vi "SQL_CloseIncidence.vi"(0 "ConnectionDSN":string, 1 "TableName":string, 2 "IncidenceID":string, 3 "ToolCribFolio":string, 4 "EWOFolio":string, 5 "Comments":string) -> ()   [LabVIEW 2017]
uses:
  <vilib>/addons/database/Connection.llb/DB Tools Open Connec (String).vi
  <vilib>/addons/database/Connection.llb/Conn Execute.vi
  <vilib>/addons/database/Recordset.llb/Rec Fetch Recordset Data (R).vi
  <vilib>/addons/database/_DB Variant To Data/Database Variant To Data.xnode
  <vilib>/addons/database/NI_Database_API.lvlib
panel:
  out "error out":errorcluster
  # "This VI Updates the hour when the machine starts production and records the downtime in minutes\ninto the database"
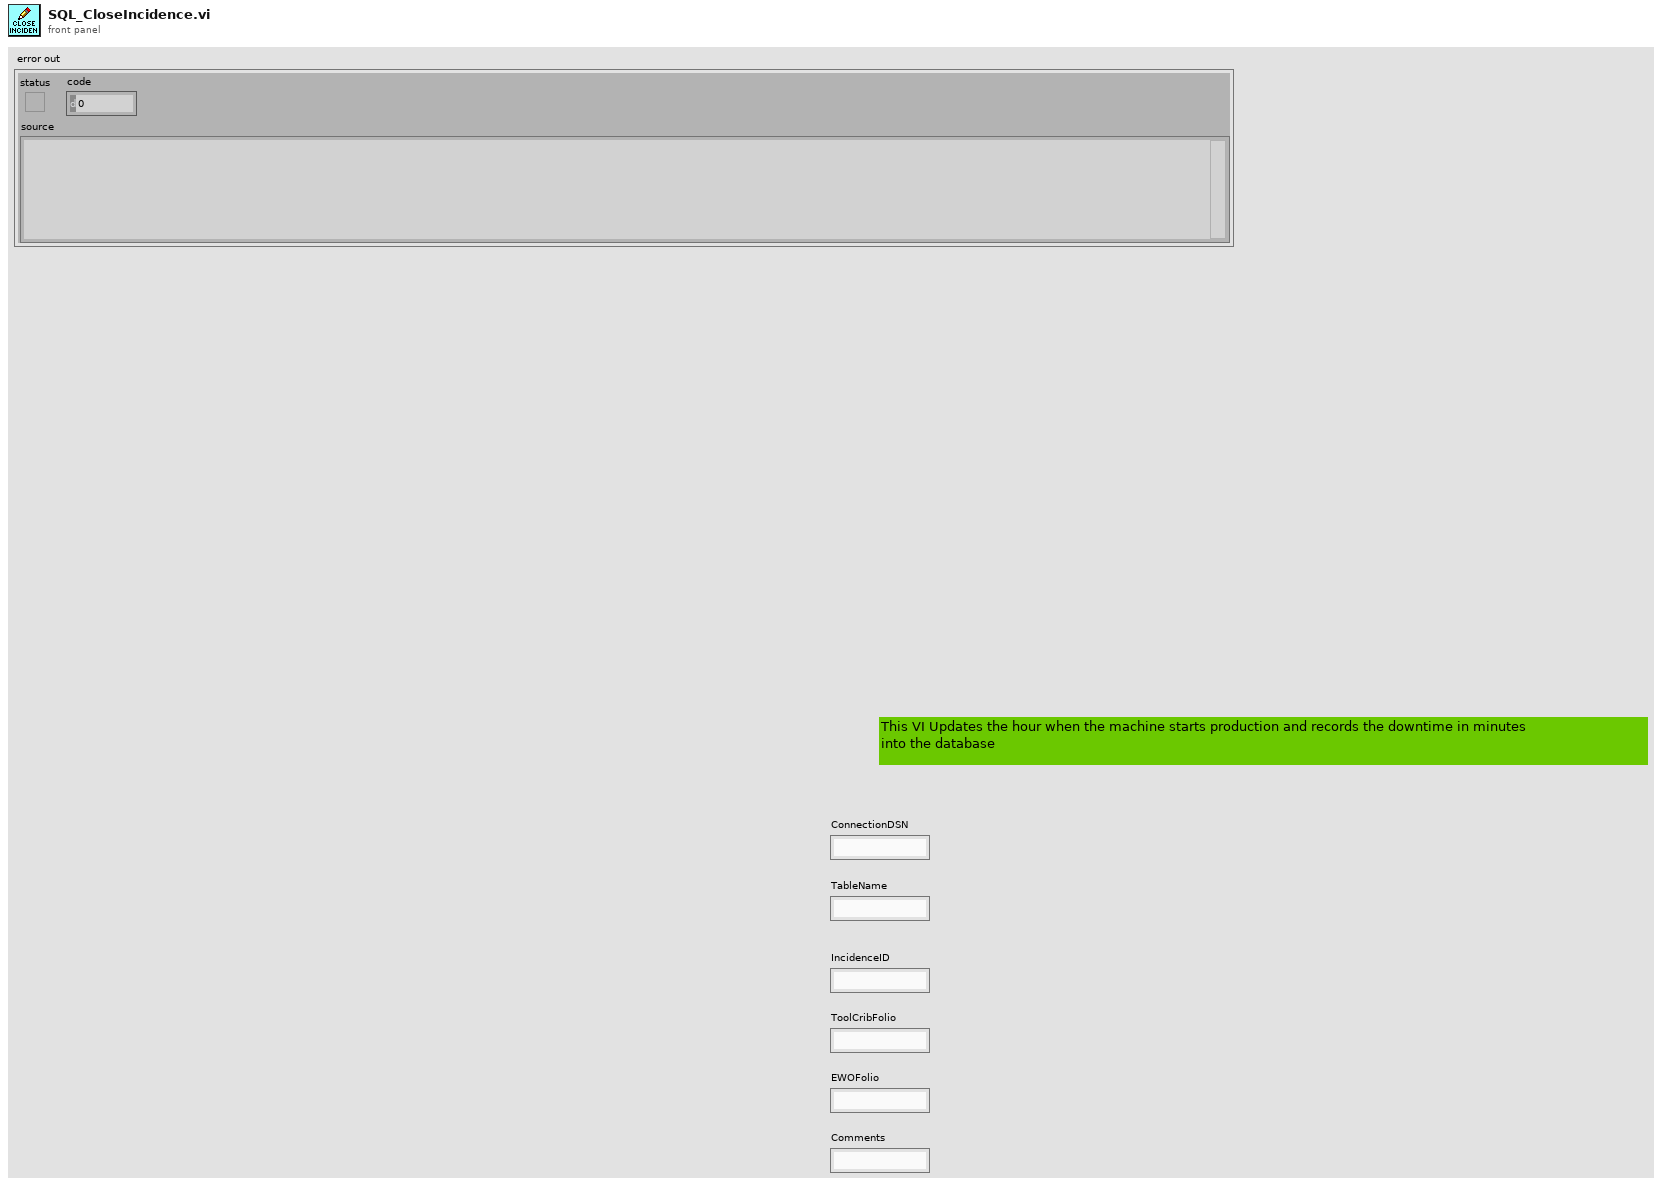
[diagram p1: front panel]
types:
  T1 = typedef "NI_Database_API.lvlib/Conn ObjectReference.ctl" = refnum<k1>
  T2 = typedef "NI_Database_API.lvlib/Rec ObjectReference.ctl" = refnum<k1>
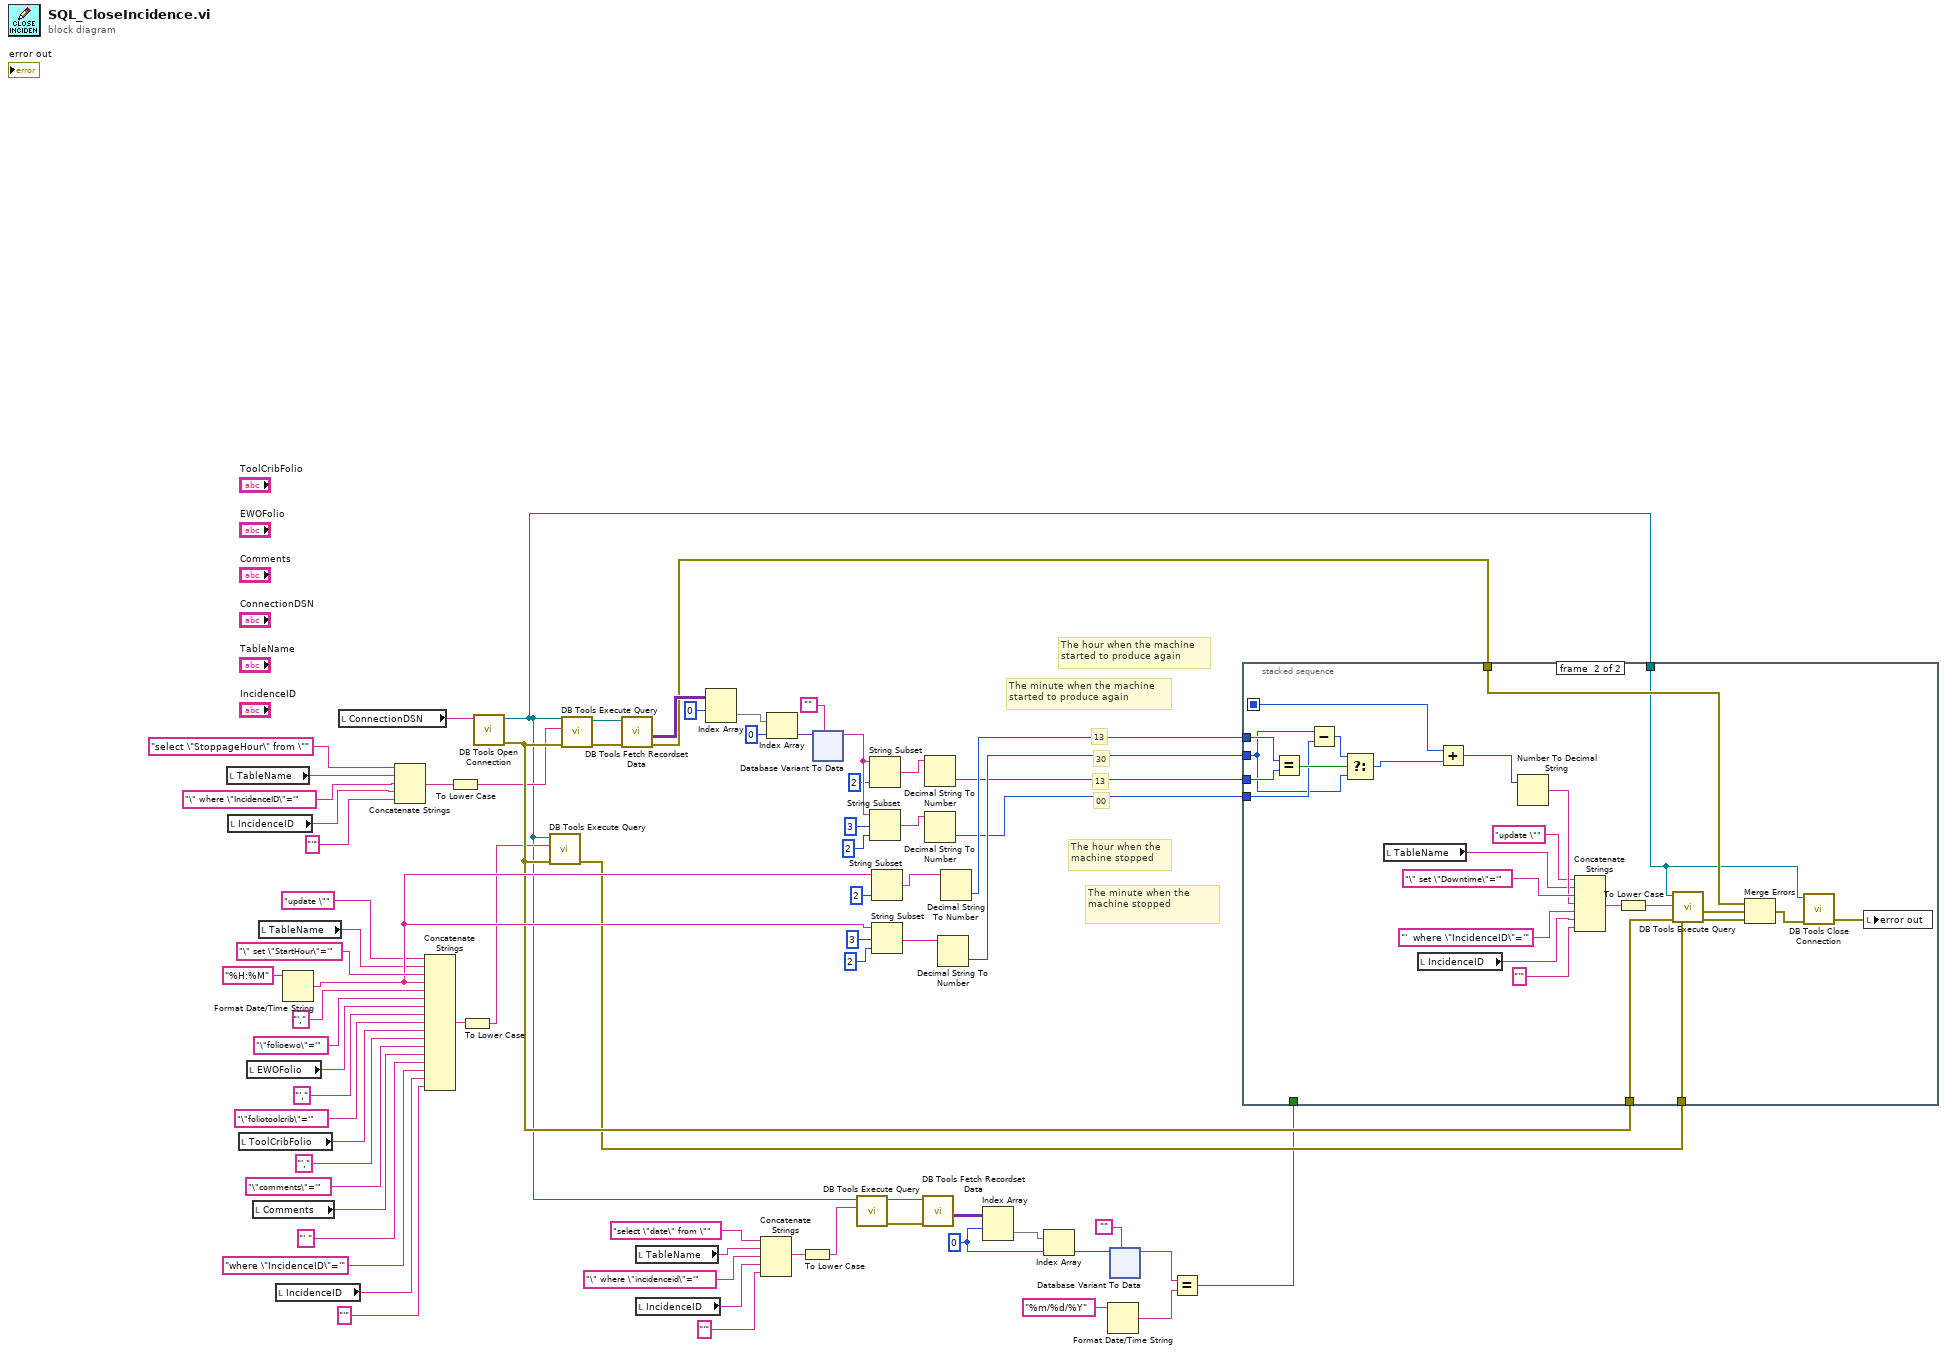
[diagram p0: block diagram]
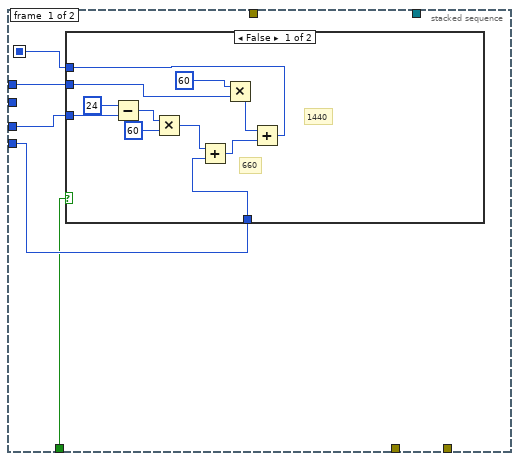
[diagram p2: hidden frame]
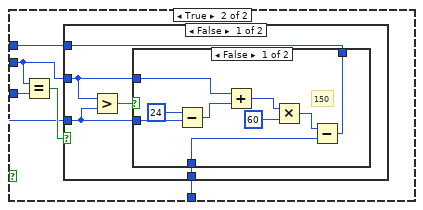
[diagram p3: hidden frame]
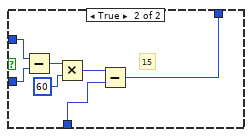
[diagram p4: hidden frame]
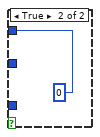
[diagram p5: hidden frame]
diagram:
  w7 = 0 ("index (row)")
  # "The hour when the machine\nstarted to produce again"
  # "The minute when the machine\nstarted to produce again"
  # "The minute when the\nmachine stopped"
  # "The hour when the\nmachine stopped"
  # "30"
  # "13"
  # "13"
  # "00"
  n1 = local read "TableName"() -> (w40:string)
  n2 = local read "IncidenceID"() -> (w38:string)
  n3 = local read "ToolCribFolio"() -> (w31:string)
  n4 = local read "EWOFolio"() -> (w33:string)
  n5 = local read "Comments"() -> (w28:string)
  n6 = local read "TableName"() -> (w43:string)
  n7 = local read "IncidenceID"() -> (w25:string)
  n8 = Format Date/Time String(time format string (%c)="%H:%M") -> (date/time string=w56:string)  [unwired: 2 in]
  n9 = local read "ConnectionDSN"() -> (w42:string)
  n10 = Concatenate Strings("select \"StoppageHour\" from \"" ("SQL query"), w40, "\" where \"IncidenceID\"='" ("SQL query"), w38, "'" ("SQL query")) -> (w21:string)
  n11 = Concatenate Strings("update \"" ("SQL query"), w43, "\" set \"StartHour\"='" ("SQL query"), w56, "',", "\"folioewo\"='" ("SQL query"), w33, "',", "\"foliotoolcrib\"='" ("SQL query"), w31, "',", "\"comments\"='" ("SQL query"), w28, "' ", "where \"IncidenceID\"='", w25, "'") -> (w23:string)
  n12 = To Lower Case(string=w21) -> (all lower case string=w20:string)
  n13 = To Lower Case(string=w23) -> (all lower case string=w22:string)
  n14 = call-poly <vilib>:"DB Tools Open Connection.vi"("connection information"=w42) -> ("error out"=w47:errorcluster, "connection reference"=w19:T1)  [unwired: 7 in]
  n15 = call-poly <vilib>:"DB Tools Execute Query.vi"("error in (no error)"=w47, "SQL query"=w22, "connection reference"=w19) -> ("error out"=w46:errorcluster)  [unwired: 5 in, 1 out]
  n16 = call-poly <vilib>:"DB Tools Execute Query.vi"("error in (no error)"=w47, "SQL query"=w20, "connection reference"=w19) -> ("error out"=w73:errorcluster, "recordset reference"=w72:T2)  [unwired: 5 in]
  n17 = call-poly <vilib>:"DB Tools Fetch Recordset Data.vi"("error in (no error)"=w73, "recordset reference"=w72) -> ("error out"=w45:errorcluster, "recordset data"=w68:variant[][])  [unwired: 3 in, 1 out]
  n18 = local read "TableName"() -> (w17:string)
  n19 = local read "IncidenceID"() -> (w15:string)
  n20 = Index Array(array=w68, index (row)=0) -> (element=w70:variant[])  [unwired: 1 in]
  n21 = Concatenate Strings("select \"date\" from \"", w17, "\" where \"incidenceid\"='", w15, "'") -> (w13:string)
  n22 = Index Array(array=w70, index=0) -> (element=w67:variant)
  n23 = To Lower Case(string=w13) -> (all lower case string=w12:string)
  n24 = xnode "Database Variant To Data"("database variant"=w67, "type"="") -> ("data"=w65:string)  [unwired: 1 in, 1 out]
  n25 = call-poly <vilib>:"DB Tools Execute Query.vi"("SQL query"=w12, "connection reference"=w19) -> ("error out"=w10:errorcluster, "recordset reference"=w11:T2)  [unwired: 6 in]
  n26 = String Subset(string=w65, length (rest)=2 ("length (rest)")) -> (substring=w51:string)  [unwired: 1 in]
  n27 = String Subset(string=w65, offset (0)=3 ("length (rest)"), length (rest)=2 ("length (rest)")) -> (substring=w50:string)
  n28 = String Subset(string=w56, length (rest)=2 ("length (rest)")) -> (substring=w55:string)  [unwired: 1 in]
  n29 = String Subset(string=w56, offset (0)=3 ("length (rest)"), length (rest)=2 ("length (rest)")) -> (substring=w53:string)
  n30 = call-poly <vilib>:"DB Tools Fetch Recordset Data.vi"("error in (no error)"=w10, "recordset reference"=w11) -> ("recordset data"=w9:variant[][])  [unwired: 3 in, 2 out]
  n31 = Decimal String To Number(string=w51) -> (number=w49:i32)  [unwired: 2 in, 1 out]
  n32 = Decimal String To Number(string=w50) -> (number=w48:i32)  [unwired: 2 in, 1 out]
  n33 = Decimal String To Number(string=w53) -> (number=w52:i32)  [unwired: 2 in, 1 out]
  n34 = Decimal String To Number(string=w55) -> (number=w54:i32)  [unwired: 2 in, 1 out]
  n35 = Index Array(array=w9, index (row)=w7) -> (element=w8:variant[])  [unwired: 1 in]
  n36 = Index Array(array=w8, index=w7) -> (element=w6:variant)
  n37 = Format Date/Time String(time format string (%c)="%m/%d/%Y") -> (date/time string=w2:string)  [unwired: 2 in]
  n38 = xnode "Database Variant To Data"("database variant"=w6, "type"="") -> ("data"=w3:string)  [unwired: 1 in, 1 out]
  n39 = Equal?(x=w3, y=w2) -> (x = y?=w1:bool)
  n40 = stacked-sequence {
    seq-local: [w78 _] -> [_ w141]
    tunnel: w52 -> [_ w118]
    tunnel: w48 -> [w75 w119]
    tunnel: w54 -> [w77 w123]
    tunnel: w49 -> [w76 w122]
    tunnel: w47 -> [_ w137]
    tunnel: w46 -> [_ w135]
    tunnel: w45 -> [_ w134]
    tunnel: w19 -> [_ w130]
    tunnel: w1 -> [w74 _]
    frame #0 {
      n41 = case shown="False" w74 {
        tunnel: [w79 w93] -> w78
        tunnel: w77 -> [w83 w92]
        tunnel: w76 -> [w89 w91]
        tunnel: w75 -> [w85 w90]
        frame False {
          # "1440"
          # "660"
          n42 = Subtract(x=24, y=w89) -> (x-y=w87:i32)
          n43 = Multiply(x=w87, y=60) -> (x*y=w84:i32)
          n44 = Add(x=w84, y=w85) -> (x+y=w81:i32)
          n45 = Multiply(x=60 ("y"), y=w83) -> (x*y=w80:i32)
          n46 = Add(x=w80, y=w81) -> (x+y=w79:i32)
        }
        frame True {
          n47 = Equal?(x=w92, y=w91) -> (x = y?=w94:bool)
          n48 = case shown="False" w94 {
            tunnel: [w98 0] -> w93
            tunnel: w92 -> [w97 _]
            tunnel: w91 -> [w96 _]
            tunnel: w90 -> [w99 _]
            frame False {
              n49 = Greater?(x=w97, y=w96) -> (0:w95:bool)
              n50 = case shown="False" w95 {
                tunnel: w97 -> [w105 w115]
                tunnel: w96 -> [w108 w114]
                tunnel: w99 -> [w102 w110]
                tunnel: [w100 w109] -> w98
                frame False {
                  # "150"
                  n51 = Subtract(x=24, y=w108) -> (x-y=w106:i32)
                  n52 = Add(x=w105, y=w106) -> (x+y=w104:i32)
                  n53 = Multiply(x=w104, y=60) -> (x*y=w101:i32)
                  n54 = Subtract(x=w101, y=w102) -> (x-y=w100:i32)
                }
                frame True {
                  # "15"
                  n55 = Subtract(x=w115, y=w114) -> (x-y=w113:i32)
                  n56 = Multiply(x=w113, y=60) -> (x*y=w111:i32)
                  n57 = Subtract(x=w111, y=w110) -> (x-y=w109:i32)
                }
              }
            }
            frame True {
            }
          }
        }
      }
    }
    frame #1 {
      n58 = Equal?(x=w123, y=w122) -> (x = y?=w121:bool)
      n59 = Subtract(x=w118, y=w119) -> (x-y=w117:i32)
      n60 = Select(t=w117, s=w121, f=w118) -> (s? t:f=w120:i32)
      n61 = local read "TableName"() -> (w129:string)
      n62 = local read "IncidenceID"() -> (w126:string)
      n63 = Add(x=w141, y=w120) -> (x+y=w131:i32)
      n64 = Number To Decimal String(number=w131) -> (decimal integer string=w139:string)  [unwired: 1 in]
      n65 = Concatenate Strings("update \"" ("SQL query"), w129, "\" set \"Downtime\"='" ("SQL query"), w139, "'  where \"IncidenceID\"='", w126, "'") -> (w124:string)
      n66 = To Lower Case(string=w124) -> (all lower case string=w125:string)
      n67 = call-poly <vilib>:"DB Tools Execute Query.vi"("error in (no error)"=w137, "SQL query"=w125, "connection reference"=w130) -> ("error out"=w136:errorcluster)  [unwired: 5 in, 1 out]
      n68 = Merge Errors(w134, w135, w136) -> (w133:errorcluster)
      n69 = call <vilib>:"DB Tools Close Connection.vi"("error in (no error)"=w133, "connection reference"=w130) -> ("error out"=w132:errorcluster)  [unwired: 5 in]
      n70 = local write "error out"(w132) -> ()
    }
  }
